vi "Request ID.vi"(11 "ErrorHandler MsgPack in":refnum<class "ErrorHandler MsgPack.lvclass">) -> (2 "Request ID":u64, 3 "ErrorHandler MsgPack out":refnum<class "ErrorHandler MsgPack.lvclass">)   [LabVIEW 2020, in "wamplv.lvlib" / "ErrorHandler MsgPack.lvclass"]
uses:
  ErrorHandler MsgPack.lvclass
  ErrorHandler MsgPack.lvclass/ErrorHandler MsgPack.ctl
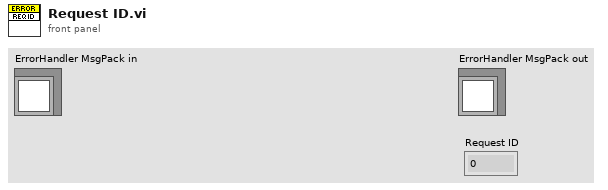
[diagram p1: front panel]
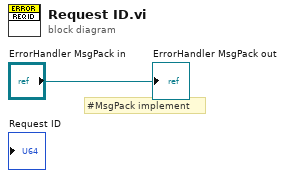
[diagram p0: block diagram]
diagram:
  # "#MsgPack implement"
  "ErrorHandler MsgPack out" <- "ErrorHandler MsgPack in"
